vi "To More Specific Type (Numeric).vi"(8 "error in (no error)":errorcluster, 11 "JSON Datatype in":refnum<class "JSON Datatype.lvclass">) -> (0 "error out":errorcluster, 3 "JSON Datatype out":refnum<class "JSON Numeric.lvclass">)   [LabVIEW 2015, in "LVJSON.lvlib" / "JSON Datatype.lvclass"]
uses:
  JSON Datatype.lvclass
  JSON Numeric/JSON Numeric.lvclass
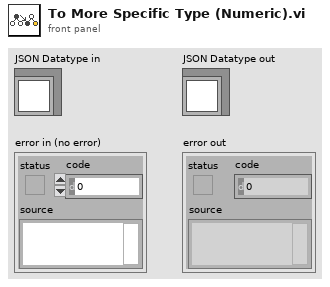
[diagram p1: front panel]
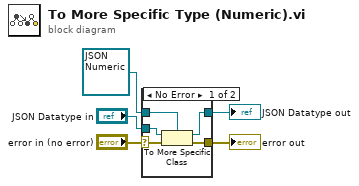
[diagram p0: block diagram]
diagram:
  n1 = case shown="No Error" "error in (no error)" {
    selector: "error in (no error)" -> [w9 w12]
    tunnel: [w8 w12] -> w4
    tunnel: [w10 w11] -> w2
    tunnel: "JSON Datatype in" -> [w6 _]
    tunnel: refnum<class "JSON Numeric.lvclass"> refnum ("target class") -> [w7 w11]
    frame No Error {
      n2 = To More Specific Class(target class=w7, reference=w6, error in=w9) -> (specific class reference=w10:refnum<class "JSON Numeric.lvclass">, error out=w8:errorcluster)
    }
    frame Error {
    }
  }
  "error out" <- w4
  "JSON Datatype out" <- w2
